vi "Assert To Report Entry.vi"(8 "error in (no error)":errorcluster, 10 "Assert":T1, 11 "Basic Test Manager in":refnum<class "Basic Test Manager.lvclass">) -> (0 "error out":errorcluster, 2 "String":string, 3 "Basic Test Manager out":refnum<class "Basic Test Manager.lvclass">)   [LabVIEW 2009, in "Caraya.lvlib" / "Basic Test Manager.lvclass"]
uses:
  Basic Test Manager.lvclass
  Assert Event Data.ctl
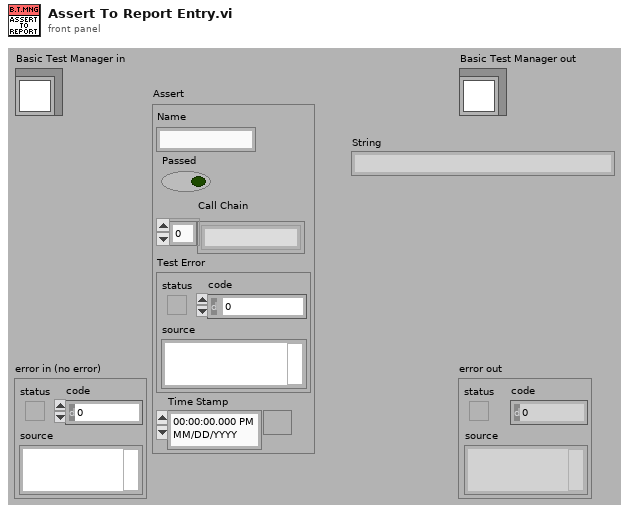
[diagram p1: front panel]
types:
  T1 = typedef "Caraya.lvlib/Basic Test Manager.lvclass/Assert Event Data.ctl" = cluster{"Name":string, "Passed":bool, "Call Chain":string[], "Test Error":errorcluster, "Time Stamp":timestamp}
  T2 = typedef "Caraya.lvlib/Basic Test Manager.lvclass/Test State.ctl" = enum16{"Empty", "Unknown", "Fail", "Pass", "Skip", "Error"}
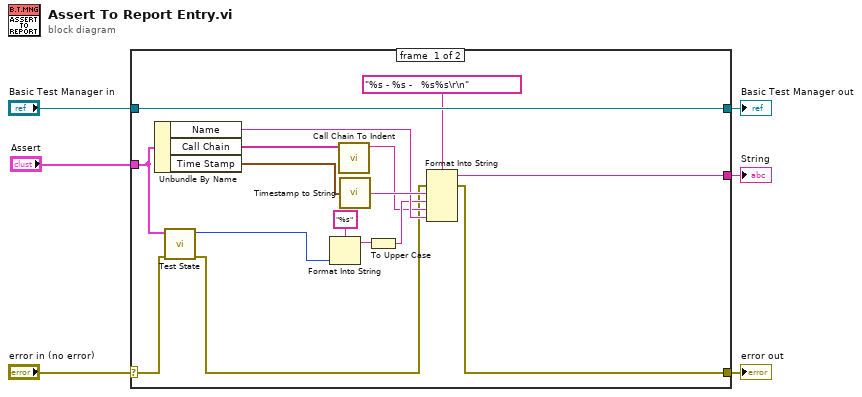
[diagram p0: block diagram]
diagram:
  n1 = case shown="No Error" "error in (no error)" {
    selector: "error in (no error)" -> [w9 w24]
    tunnel: [w17 w24] -> w5
    tunnel: [w22 w23] -> w3
    tunnel: "Basic Test Manager in" -> [w22 w23]
    tunnel: "Assert" -> [w11 _]
    tunnel: [w16 _] -> w1
    frame #0 {
      n2 = Unbundle By Name(w11) -> ("Name"=w18:string, "Call Chain"=w7:string[], "Time Stamp"=w21:timestamp)
      n3 = call "Test State.vi"("error in (no error)"=w9, "Test Event"=w11) -> ("error out"=w8:errorcluster, "Test State"=w10:T2)  [unwired: 8 in]
      n4 = Format Into String(format string="%s", w10) -> (resulting string=w14:string)  [unwired: 2 in, 1 out]
      n5 = call "Call Chain To Indent.vi"("Call Chain"=w7) -> ("Indent"=w12:string)  [unwired: 10 in]
      n6 = call "Timestamp to String.vi"("Time Stamp"=w21) -> ("date/time string"=w20:string)
      n7 = To Upper Case(1:w14) -> (0:w13:string)
      n8 = Format Into String(format string="%s - %s -   %s%s\r\n", error in=w8, w20, w13, w12, w18) -> (resulting string=w16:string, error out=w17:errorcluster)  [unwired: 1 in]
    }
    frame #1 {
    }
  }
  "error out" <- w5
  "Basic Test Manager out" <- w3
  "String" <- w1
